vi "ChirpOOPV3.vi"() -> ()   [LabVIEW 2014, in "ChirpV2.lvclass"]
uses:
  ChirpV2.lvclass
  StateV2.ctl
panel:
  out "#left":i32
  out "?":dbl(slide) scale=0.0..1.0
  out "size(s)":i32
  out "Experiment Variables":T2={"DC_Bias"=0.0, "StartFreq"=0.0, "Duration"=0.0, "State"=enum."Initialization", "window ratio"=0.0, "Final Freq"=0.0}
  out "output cluster":T2={"DC_Bias"=0.0, "StartFreq"=0.0, "Duration"=0.0, "State"=enum."Initialization", "window ratio"=0.0, "Final Freq"=0.0}
  in  "R external(Ohm)":dbl=33.0
  out "error out":errorcluster
  out "Waveform Graph":dynamicdata(graph)
  in  "Path":path=path "C:/Users/YuanYuan/Desktop/Labview Data/Database"
  in  "Sample Name":string="TOKIN1"
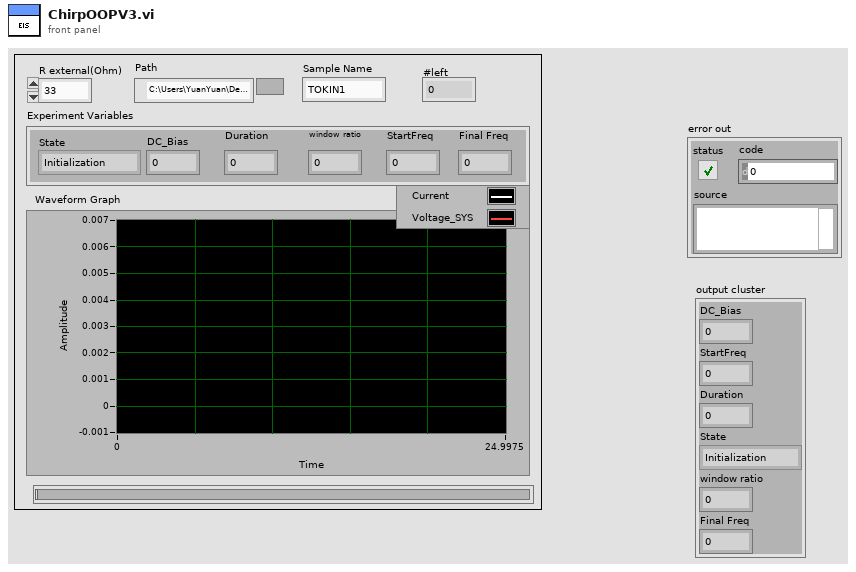
[diagram p1: front panel]
types:
  T1 = typedef "ChirpV2.lvclass/StateV2.ctl" = enum16{"WaitDC", "Initialization", "ChirpSetUp", "Wait", "ChirpMeasurement", "DFT", "WriteData", "Queue", "Ternimation"}
  T2 = cluster{"DC_Bias":dbl, "StartFreq":dbl, "Duration":dbl, "State":T1, "window ratio":dbl, "Final Freq":dbl}
  T3 = cluster{"T":dbl, "Fst":dbl, "Fends":dbl, "Dc":dbl, "w ratio":dbl}
  T4 = cluster{"T":dbl, "Fst":dbl, "Fends":dbl, "Dc":dbl, "w ratio":dbl}[]
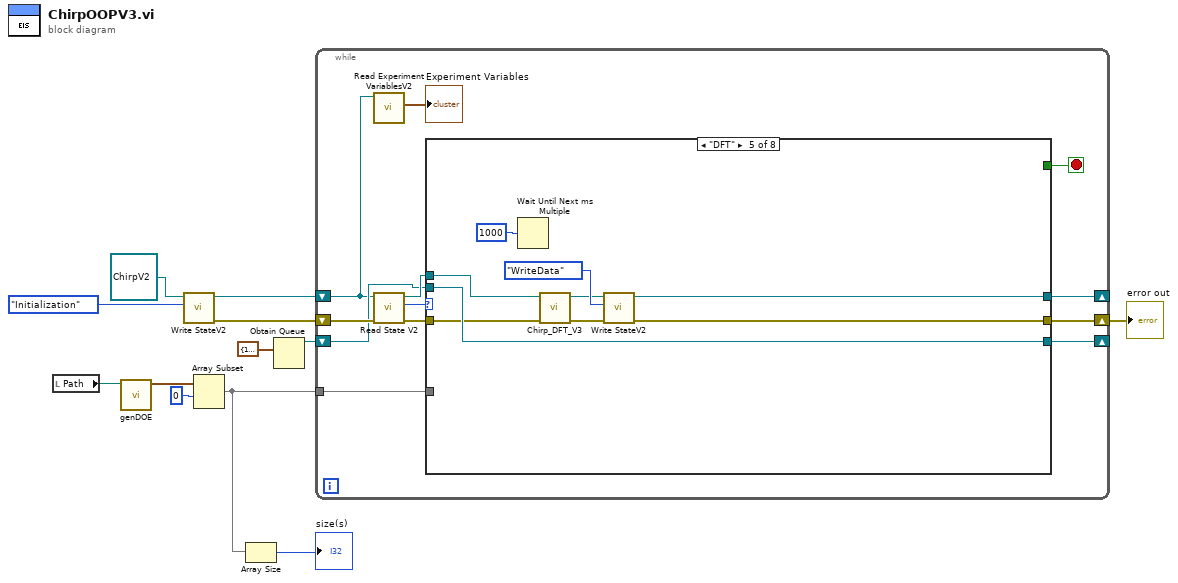
[diagram p0: block diagram]
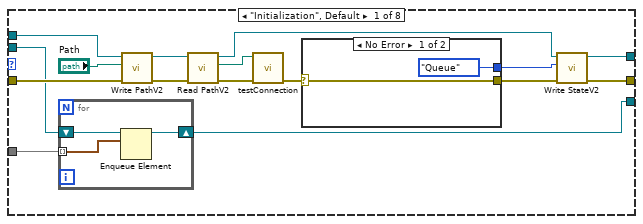
[diagram p2: hidden frame]
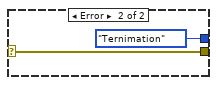
[diagram p3: hidden frame]
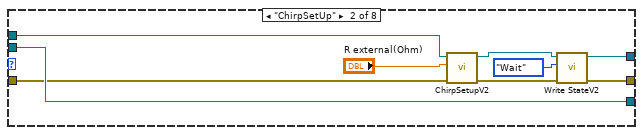
[diagram p4: hidden frame]
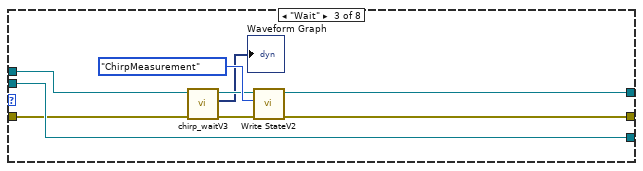
[diagram p5: hidden frame]
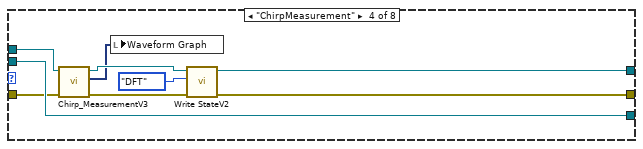
[diagram p6: hidden frame]
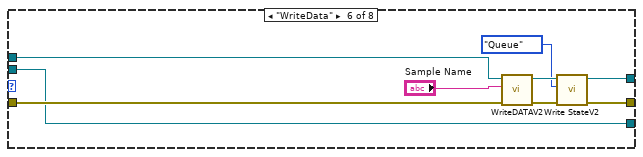
[diagram p7: hidden frame]
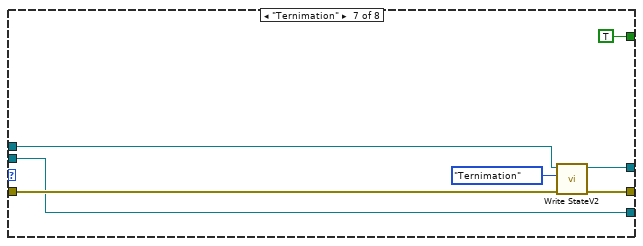
[diagram p8: hidden frame]
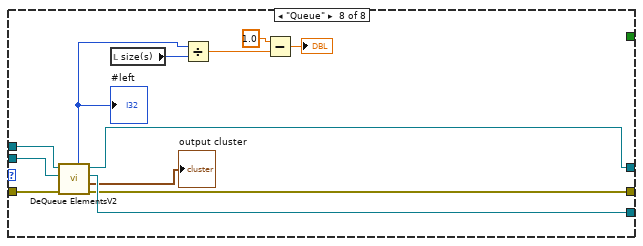
[diagram p9: hidden frame]
diagram:
  n1 = local read "Path"() -> (w5:path)
  n2 = call "genDOE.vi"("db_File"=w5) -> ("Array 2"=w4:T4)  [unwired: 9 in, 1 out]
  n3 = call-dynamic "Write StateV2.vi"("Enum"=StateV2."Initialization", "ChirpV2 in"=refnum<class "ChirpV2.lvclass"> refnum ("ChirpV2.lvclass")) -> ("error out"=w9:errorcluster, "ChirpV2 out"=w10:refnum<class "ChirpV2.lvclass">)  [unwired: 8 in]
  n4 = Array Subset(array=w4, index=0) -> (w3:T4)  [unwired: 1 in]
  n5 = Array Size(array=w3) -> (size(s)=→"size(s)":i32)
  n6 = Obtain Queue(element data type=T3 {"T"=1010.0, "Fst"=0.001, "Fends"=10.0, "Dc"=0.001, "w ratio"=0.001} ("DOE parameters 2")) -> (queue out=w7:refnum<queue>)  [unwired: 4 in, 2 out]
  n7 = while {
    shift-right: [w23] -> _
    shift-left: w10 -> [w14]
    shift-right: [w19] -> w8
    shift-left: w9 -> [w21]
    shift-right: [w16] -> _
    shift-left: w7 -> [w17]
    tunnel: w3 -> [w15]
    stop <- w18 stop-if-true
    n8 = call-dynamic "Read Experiment VariablesV2.vi"("ChirpV2 in"=w14) -> ("Experiment Variables"=→"Experiment Variables":T2)  [unwired: 8 in, 2 out]
    n9 = call-dynamic "Read State V2.vi"("error in (no error)"=w21, "ChirpV2 in"=w14) -> ("error out"=w20:errorcluster, "Enum"=w24:T1, "ChirpV2 out"=w22:refnum<class "ChirpV2.lvclass">)  [unwired: 7 in]
    n10 = case shown="\"DFT\"" w24 {
      tunnel: [w39 w53 w63 w73 w81 w87 w98 w107] -> w23
      tunnel: w22 -> [w38 w56 w61 w70 w78 w85 w96 w110]
      tunnel: w20 -> [w37 w48 w60 w69 w77 w92 w95 w109]
      tunnel: [w34 w52 w65 w74 w80 w88 w97 w106] -> w19
      tunnel: [_ _ _ _ _ _ TRUE _] -> w18
      tunnel: w17 -> [w27 w50 w62 w71 w79 w84 w93 w111]
      tunnel: [w26 w50 w62 w71 w79 w84 w93 w108] -> w16
      tunnel: w15 -> [w25 _ _ _ _ _ _ _]
      frame "Initialization", Default {
        n11 = for {
          shift-right: [w42] -> w26
          shift-left: w27 -> [w43]
          tunnel: w25 -> [w41] mode=indexing
          n12 = Enqueue Element(queue=w43, element=w41) -> (queue out=w42:refnum<queue>)  [unwired: 2 in, 2 out]
        }
        n13 = call-dynamic "Write PathV2.vi"("error in (no error)"=w37, "Path"="Path", "ChirpV2 in"=w38) -> ("error out"=w30:errorcluster, "ChirpV2 out"=w32:refnum<class "ChirpV2.lvclass">)  [unwired: 7 in]
        n14 = call-dynamic "Read PathV2.vi"("error in (no error)"=w30, "ChirpV2 in"=w32) -> ("error out"=w29:errorcluster, "Path"=w28:path, "ChirpV2 out"=w31:refnum<class "ChirpV2.lvclass">)  [unwired: 7 in]
        n15 = call "testConnection.vi"("error in (no error)"=w29, "db_File"=w28) -> ("error out"=w35:errorcluster)  [unwired: 9 in]
        n16 = case shown="No Error" w35 {
          selector: w35 -> [w44 w46]
          tunnel: [StateV2."Queue" ("Enum") StateV2."Ternimation" ("Enum")] -> w40
          tunnel: [w44 w46] -> w33
          frame No Error {
          }
          frame Error {
          }
        }
        n17 = call-dynamic "Write StateV2.vi"("error in (no error)"=w33, "Enum"=w40, "ChirpV2 in"=w31) -> ("error out"=w34:errorcluster, "ChirpV2 out"=w39:refnum<class "ChirpV2.lvclass">)  [unwired: 7 in]
      }
      frame "ChirpSetUp" {
        n18 = call "ChirpSetupV2.vi"("error in (no error)"=w48, "R external(Ohm)"="R external(Ohm)", "ChirpV2 in"=w56) -> ("error out"=w54:errorcluster, "ChirpV2 out"=w55:refnum<class "ChirpV2.lvclass">)  [unwired: 7 in]
        n19 = call-dynamic "Write StateV2.vi"("error in (no error)"=w54, "Enum"=StateV2."Wait", "ChirpV2 in"=w55) -> ("error out"=w52:errorcluster, "ChirpV2 out"=w53:refnum<class "ChirpV2.lvclass">)  [unwired: 7 in]
      }
      frame "Wait" {
        n20 = call "chirp_waitV3.vi"("error in (no error)"=w60, "ChirpV2 in"=w61) -> ("error out"=w59:errorcluster, "data"=→"Waveform Graph":dynamicdata, "ChirpV2 out"=w58:refnum<class "ChirpV2.lvclass">)  [unwired: 7 in]
        n21 = call-dynamic "Write StateV2.vi"("error in (no error)"=w59, "Enum"=StateV2."ChirpMeasurement", "ChirpV2 in"=w58) -> ("error out"=w65:errorcluster, "ChirpV2 out"=w63:refnum<class "ChirpV2.lvclass">)  [unwired: 7 in]
      }
      frame "ChirpMeasurement" {
        n22 = call "Chirp_MeasurementV3.vi"("error in (no error) 2"=w69, "ChirpV2 in 2"=w70) -> ("error out 2"=w67:errorcluster, "data 3"=w66:dynamicdata, "ChirpV2 out 2"=w68:refnum<class "ChirpV2.lvclass">)  [unwired: 7 in]
        n23 = local write "Waveform Graph"(w66) -> ()
        n24 = call-dynamic "Write StateV2.vi"("error in (no error)"=w67, "Enum"=StateV2."DFT", "ChirpV2 in"=w68) -> ("error out"=w74:errorcluster, "ChirpV2 out"=w73:refnum<class "ChirpV2.lvclass">)  [unwired: 7 in]
      }
      frame "DFT" {
        n25 = Wait Until Next ms Multiple(millisecond multiple=u32 1000) -> ()  [unwired: 1 out]
        n26 = call "Chirp_DFT_V3.vi"("error in (no error)"=w77, "ChirpV2 in"=w78) -> ("error out"=w75:errorcluster, "ChirpV2 out"=w76:refnum<class "ChirpV2.lvclass">)  [unwired: 8 in]
        n27 = call-dynamic "Write StateV2.vi"("error in (no error)"=w75, "Enum"=StateV2."WriteData", "ChirpV2 in"=w76) -> ("error out"=w80:errorcluster, "ChirpV2 out"=w81:refnum<class "ChirpV2.lvclass">)  [unwired: 7 in]
      }
      frame "WriteData" {
        n28 = call "WriteDATAV2.vi"("error in (no error)"=w92, "Sample Name"="Sample Name", "ChirpV2 in"=w85) -> ("error out"=w89:errorcluster, "ChirpV2 out"=w90:refnum<class "ChirpV2.lvclass">)  [unwired: 7 in]
        n29 = call-dynamic "Write StateV2.vi"("error in (no error)"=w89, "Enum"=StateV2."Queue", "ChirpV2 in"=w90) -> ("error out"=w88:errorcluster, "ChirpV2 out"=w87:refnum<class "ChirpV2.lvclass">)  [unwired: 7 in]
      }
      frame "Ternimation" {
        n30 = call-dynamic "Write StateV2.vi"("error in (no error)"=w95, "Enum"=StateV2."Ternimation", "ChirpV2 in"=w96) -> ("error out"=w97:errorcluster, "ChirpV2 out"=w98:refnum<class "ChirpV2.lvclass">)  [unwired: 7 in]
      }
      frame "Queue" {
        n31 = call "DeQueue ElementsV2.vi"("error in (no error)"=w109, "queue in"=w111, "ChirpV2 in"=w110) -> ("error out"=w106:errorcluster, "output cluster"=→"output cluster":T2, "queue out"=w108:refnum<queue>, "ChirpV2 out"=w107:refnum<class "ChirpV2.lvclass">, "#left"=w104:i32)  [unwired: 4 in]
        "#left" <- w104
        n32 = local read "size(s)"() -> (w103:i32)
        n33 = Divide(x=w104, y=w103) -> (x/y=w102:dbl)
        n34 = Subtract(x=1.0, y=w102) -> (x-y=→"?":dbl)
      }
    }
  }
  "error out" <- w8
